vi "GetState.vi"(8 "error in (no error)":errorcluster) -> (0 "error out":errorcluster, 2 "State":T1)   [LabVIEW 2019, in "MainStates.lvclass"]
uses:
  MainStates.lvclass
  TypeDef/MainState.ctl
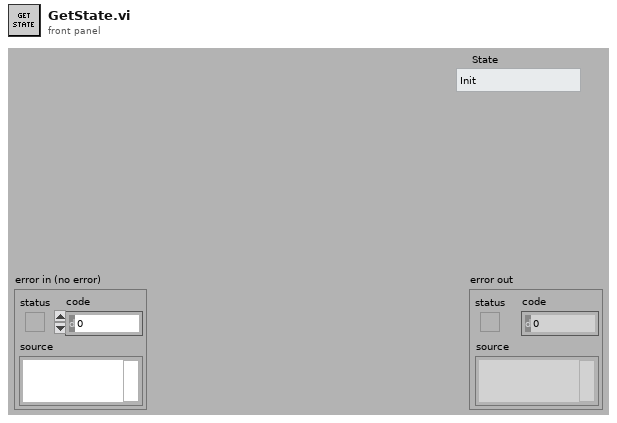
[diagram p1: front panel]
types:
  T1 = typedef "MainState.ctl" = enum16{"Init", "Idle", "Safe Stop", "Normal Working", "Critical Error", "Closing"}
  T2 = typedef "MainStates.lvclass/ObjectAttributes.ctl" = cluster{"State":T1}
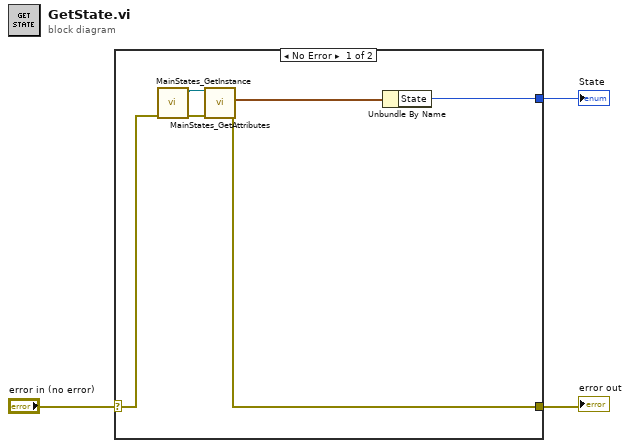
[diagram p0: block diagram]
diagram:
  n1 = case shown="No Error" "error in (no error)" {
    selector: "error in (no error)" -> [w5 w10]
    tunnel: [w8 w10] -> w2
    tunnel: [w7 _] -> w1
    frame No Error {
      n2 = call "MainStates_GetInstance.vi"("error in (no error)"=w5) -> ("error out"=w4:errorcluster, "reference out"=w6:refnum<class "MainStates.lvclass">)  [unwired: 6 in, 3 out]
      n3 = call "MainStates_GetAttributes.vi"("error in (no error)"=w4, "reference in"=w6) -> ("error out"=w8:errorcluster, "Data"=w9:T2)  [unwired: 6 in, 2 out]
      n4 = Unbundle By Name(w9) -> ("State"=w7:T1)
    }
    frame Error {
    }
  }
  "error out" <- w2
  "State" <- w1
